vi "EnFlo_Turntable_Control.vi"(3 "Mode":T5=enum."Run VI", 5 "Traverse line In":T2={"Start X"=0.0, "Start Y"=0.0, "Start Z"=0.0, "End X"=0.0, "End Y"=0.0, "End Z"=0.0, "No. of pts."=6, "Spacing"=enum."Linear", "Filename"=path "C:/Enflo_Data_Local/2015/EnFlo_Tunnel/Paul_Hayden/Calibrations/Cal_06-2015/Datum_Block_1.xls", "Tunnel Speed"=0.0, "Averaging time (min)"=0.01, "Extra Commands"="", "Carrier_1 Q (l/min)"=nan, "Carrier_2 Q (l/min)"=nan, "Trace Gas Concentration (%)"=nan, "Specific Arguments"="Datum_Image_Calibration.vi  ", "Comments"="", "Row No"=0, "Row Type Selector"=enum."Run VI Named:", "Completion time"="12:51  12-06-2015", "Row Duration (mins)"=0.11291999999999999, "No. of Valid pts."=6, "Meas Setup File"="Trav_Cam_Picture.xls"} {"Carrier_2 Q (l/min)" format="%#.2f"; "Row Duration (mins)" format="%#.1f"; "Row No" min=0; "Trace Gas Concentration (%)" min=0.0 format="%#_4f"; "Carrier_1 Q (l/min)" format="%#.2f"; "Tunnel Speed" format="%#.2f"; "Start X" format="%#.2f"; "Start Y" format="%#.2f"; "Start Z" format="%#.2f"; "End X" format="%#.2f"; "End Y" format="%#.2f"; "End Z" format="%#.2f"; "Averaging time (min)" min=0.0 format="%#.2f"}) -> (0 "Error Message":string, 1 "Status":T1, 2 "Traverse line Out":T2={"Start X"=0.0, "Start Y"=0.0, "Start Z"=0.0, "End X"=0.0, "End Y"=0.0, "End Z"=0.0, "No. of pts."=6, "Spacing"=enum."Linear", "Filename"=path "C:/Enflo_Data_Local/2015/EnFlo_Tunnel/Paul_Hayden/Calibrations/Cal_06-2015/Datum_Block_1.xls", "Tunnel Speed"=0.0, "Averaging time (min)"=0.01, "Extra Commands"="", "Carrier_1 Q (l/min)"=nan, "Carrier_2 Q (l/min)"=nan, "Trace Gas Concentration (%)"=nan, "Specific Arguments"="Datum_Image_Calibration.vi  ", "Comments"="", "Row No"=0, "Row Type Selector"=enum."Run VI Named:", "Completion time"="12:51  12-06-2015", "Row Duration (mins)"=0.11291999999999999, "No. of Valid pts."=6, "Meas Setup File"="Trav_Cam_Picture.xls"} {"Carrier_2 Q (l/min)" format="%#.2f"; "Row Duration (mins)" format="%#.1f"; "Row No" min=0; "Trace Gas Concentration (%)" min=0.0 format="%#_4f"; "Carrier_1 Q (l/min)" format="%#.2f"; "Tunnel Speed" format="%#.2f"; "Start X" format="%#.2f"; "Start Y" format="%#.2f"; "Start Z" format="%#.2f"; "End X" format="%#.2f"; "End Y" format="%#.2f"; "End Z" format="%#.2f"; "Averaging time (min)" min=0.0 format="%#.2f"})   [LabVIEW 2015]
uses:
  Gen Trav/Traverse_cluster.ctl
  Gen Trav/Spacing.ctl
  Controls/Multi_run_mode.ctl
  Controls/User_Specific_mode.ctl
  Gen Trav/Multi_Run_Status.ctl
  Gen Trav/Trav_mode.ctl
  Controls/Home.ctl
  Controls/Setup.ctl
  Controls/Save_Data.ctl
  ADAM Client/Sub VIs/ADAM Controls/Update_scan_value.ctl
  <vilib>/Analysis/baseanly.llb/Mean (DBL).vi
  Globals/Extra_Commands_Global.vi
  Globals/Trav_pos_global.vi
  Globals/Dynamic_call_global.ph.vi
  <vilib>/Analysis/NI_AALBase.lvlib
panel:
  in  "Ratio of Error to move":dbl=0.75
  in  "stop":bool
  out "Av Meas Angle":dbl format="%0.3f"
  out "Meas Angle":dbl[](array[numeric])
  out "Errors":dbl[](array[numeric])
  in  "Numeric":i32=1
  out "Error in Turntable":dbl(graph)
  in  "Angle Tolerance":dbl=0.01 format="%#_13g"
  out "Turntable Error":dbl
  out "Motor Position (Angle)":dbl(graph)
  out "Demanded Deg":dbl format="%#.4f"
  out "Correct Position":bool
  out "Drive needs relaxing?":bool
  out "Relax Drive":dbl=0.25
  out "+ve Rotation":bool
  out "Motor Current Position":dbl
  # "X           Y            Z"
  # "Start"
  # "End"
  # "X           Y            Z"
  # "Start"
  # "End"
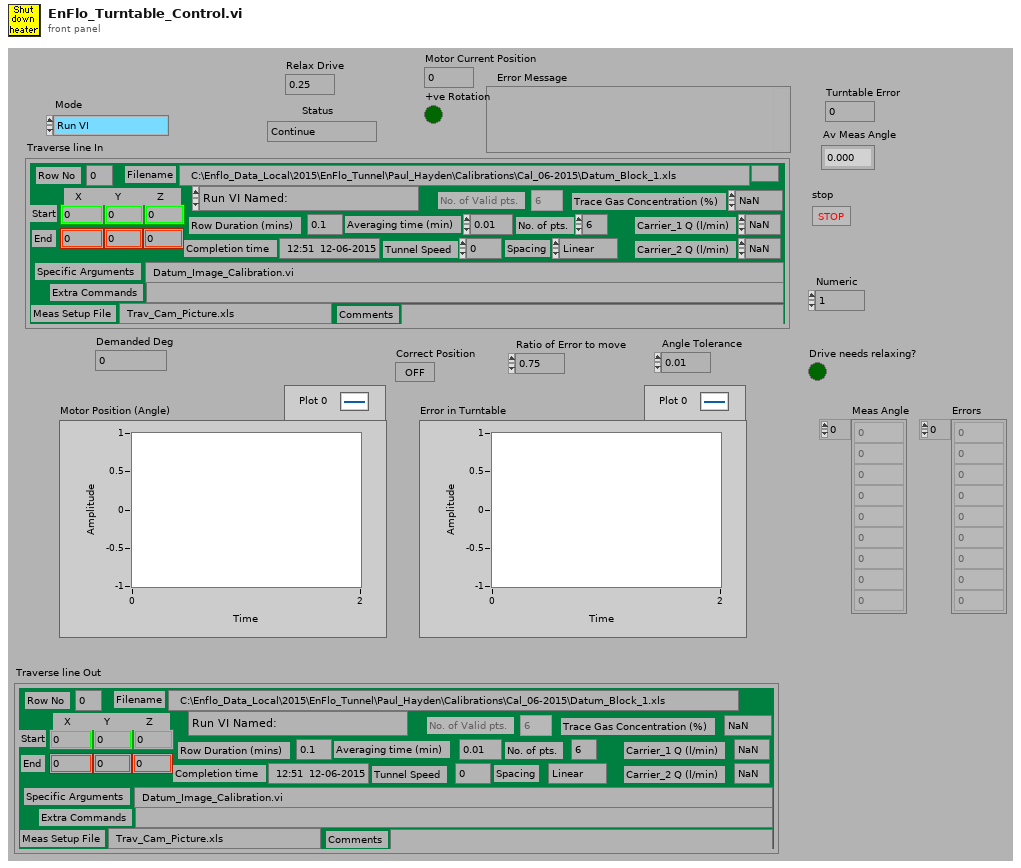
[diagram p1: front panel]
types:
  T1 = typedef "Multi_Run_Status.ctl" = enum16{"Continue", "Jump to Next Point", "Jump to Next Row", "Jump To Fall Back", "Terminate Run"}
  T2 = typedef "Traverse_cluster.ctl" = cluster{"Start X":sgl, "Start Y":sgl, "Start Z":sgl, "End X":sgl, "End Y":sgl, "End Z":sgl, "No. of pts.":i32, "Spacing":T3, "Filename":path, "Tunnel Speed":dbl, "Averaging time (min)":dbl, "Extra Commands":string, "Carrier_1 Q (l/min)":dbl, "Carrier_2 Q (l/min)":dbl, "Trace Gas Concentration (%)":dbl, "Specific Arguments":string, "Comments":string, "Row No":i32, "Row Type Selector":T4, "Completion time":string, "Row Duration (mins)":dbl, "No. of Valid pts.":i32, "Meas Setup File":string}
  T3 = typedef "Spacing.ctl" = enum16{"Linear", "Log", "Gauss", "Specified", "N/A"}
  T4 = typedef "Multi_run_mode.ctl" = enum16{"Move Traverse Only", "Set Tunnel Speed Only", "Set Source Only", "Set Measurement Conditions", "Single Measurement", "Vertical Profile", "Lateral Profile", "Longitudinal Profile", "Explore Volume", "Multi-Axis Profile", "Auto Calibrate", "Meas Fast FID Bkgnd", "Check Beam Power", "Scanning Valve Measurement", "Run VI Named:", "Set ADAM Ch", "Wait (minutes)", "Send Message", "Synchronize With:", "Fall Back to this Row", "Turn Off Row Repeating", "Blank Row", "Traverse 3D Volume"}
  T5 = typedef "User_Specific_mode.ctl" = enum16{"Check VI only", "Run VI"}
  T6 = typedef "Home.ctl" = enum16{"Don't Home", "Home  +X", "Home  -X", "Home  +Y", "Home  -Y", "Home  +Z", "Home  -Z"}
  T7 = typedef "Trav_mode.ctl" = enum16{"Move traverse", "Read traverse position", "Teach Position"}
  T8 = typedef "Save_Data.ctl" = enum16{"Save No Data", "Save Data"}
  T9 = typedef "Setup.ctl" = enum16{"Run Program", "Show Setup", "Save Current Setup", "Setup Front Panel"}
  T10 = typedef "Update_scan_value.ctl" = cluster{"Channel Name":string, "New Value":dbl}
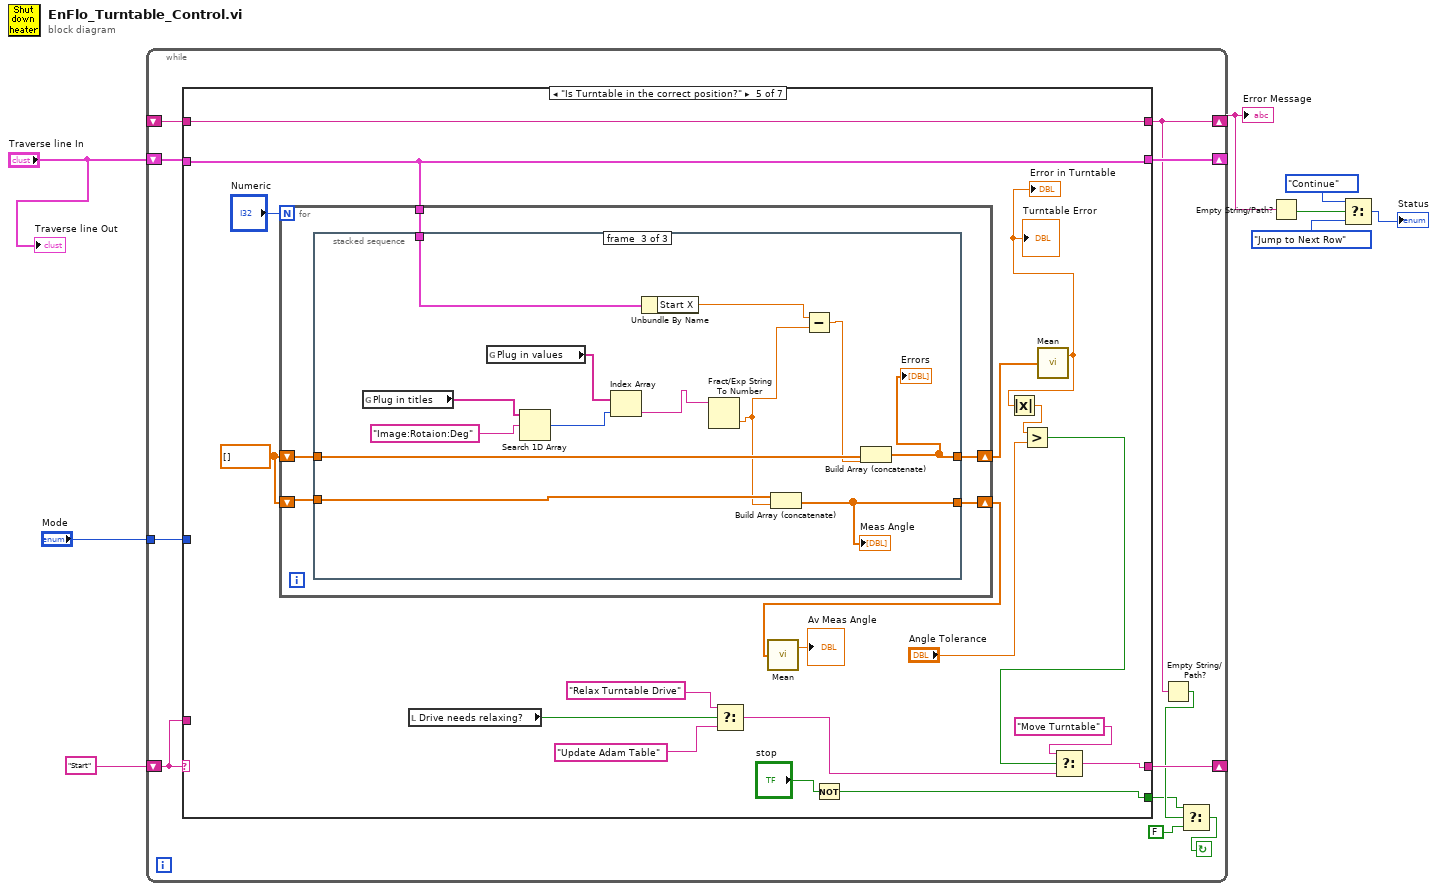
[diagram p0: block diagram]
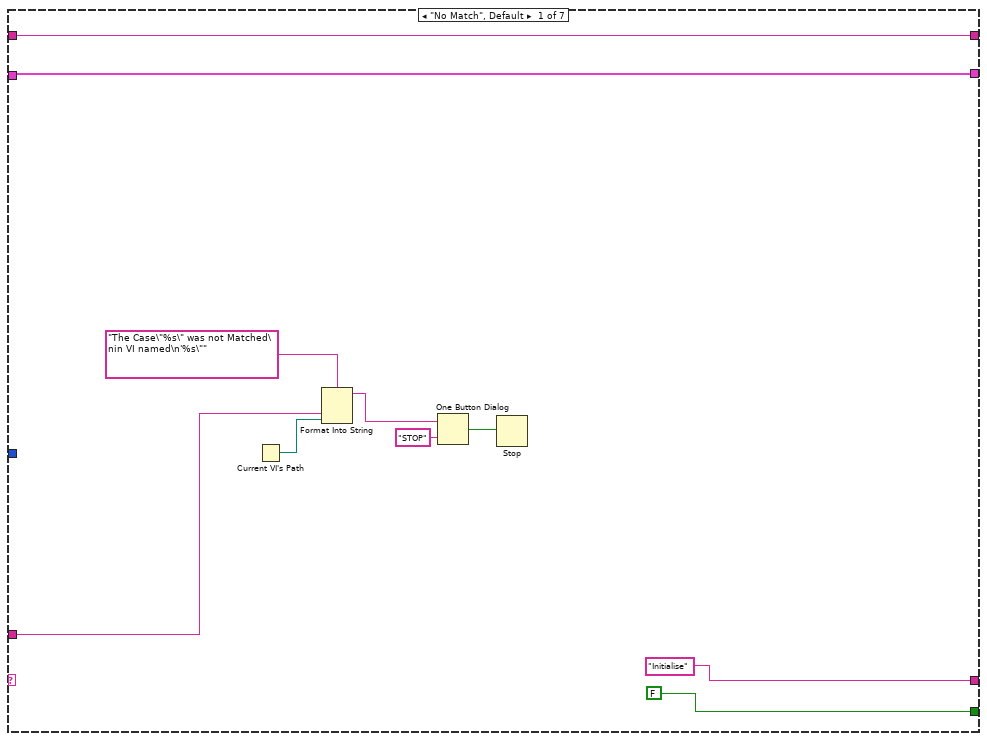
[diagram p2: hidden frame]
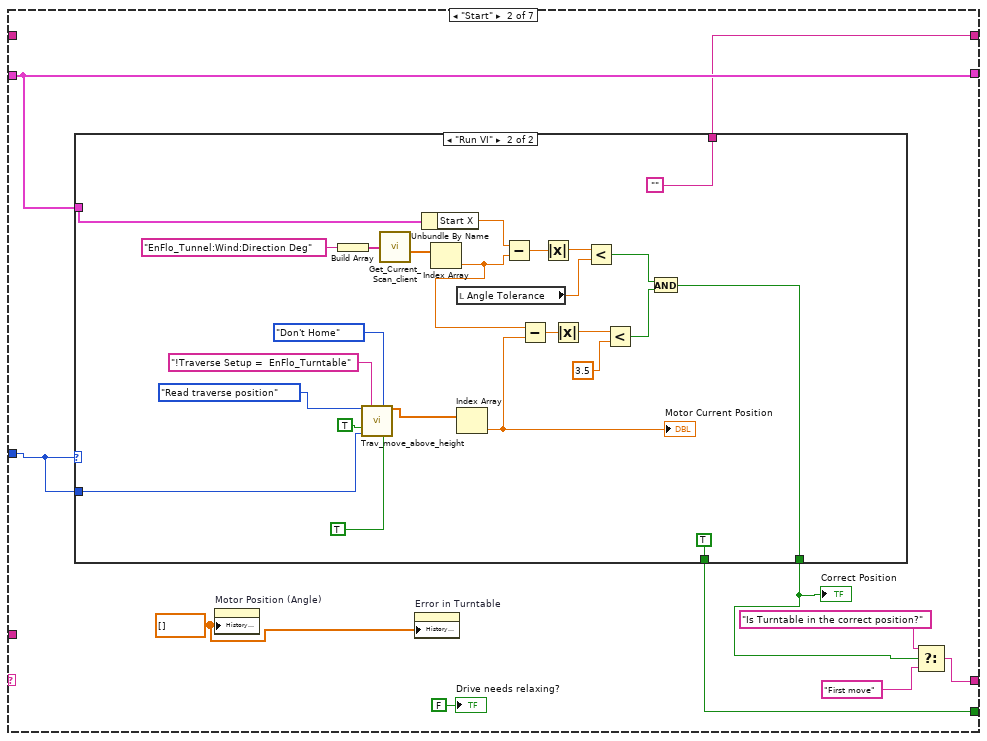
[diagram p3: hidden frame]
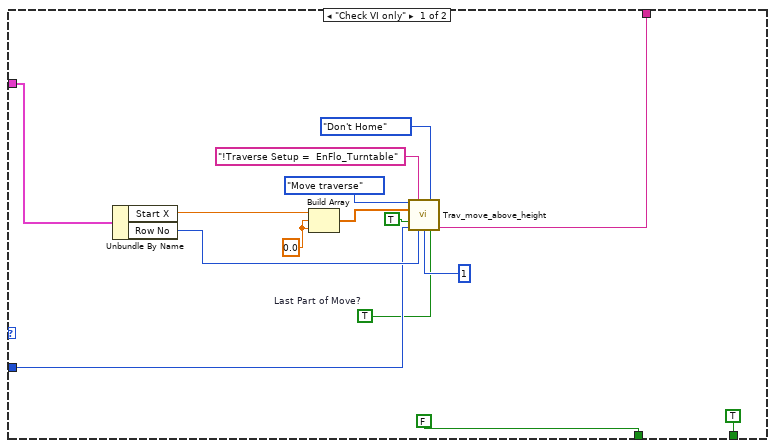
[diagram p4: hidden frame]
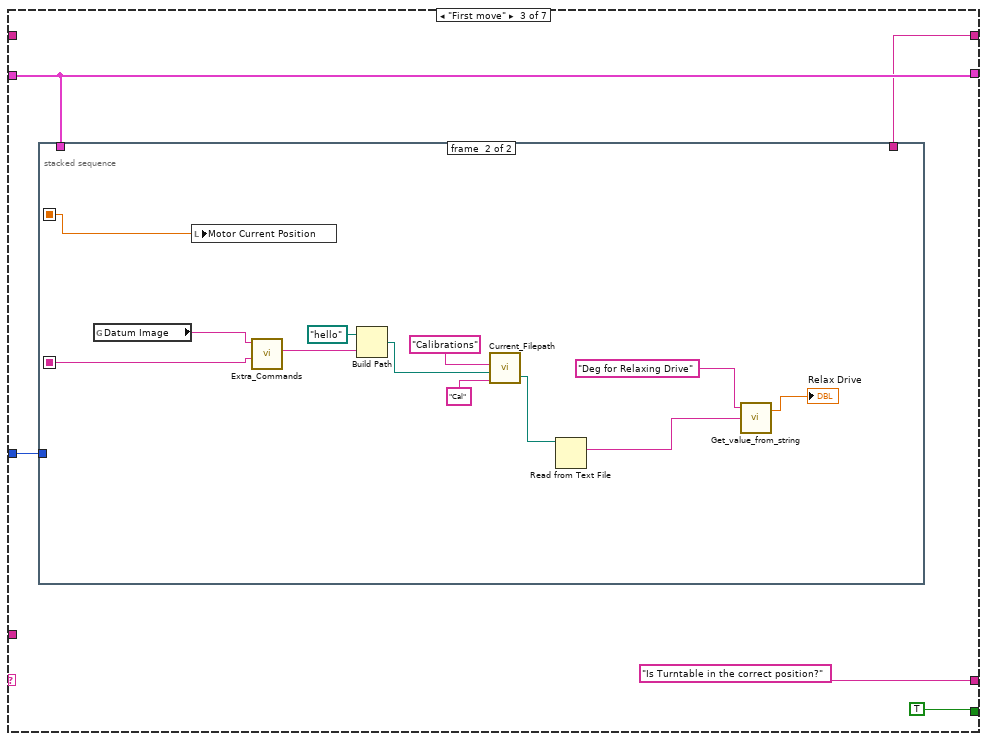
[diagram p5: hidden frame]
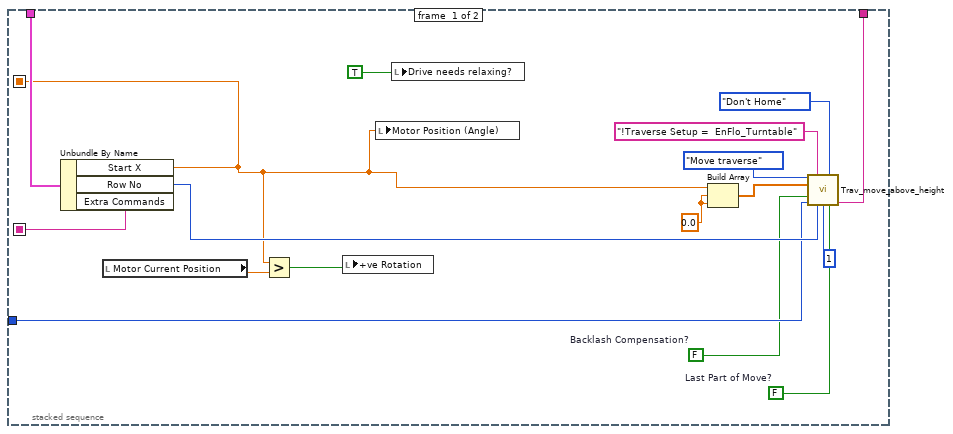
[diagram p6: hidden frame]
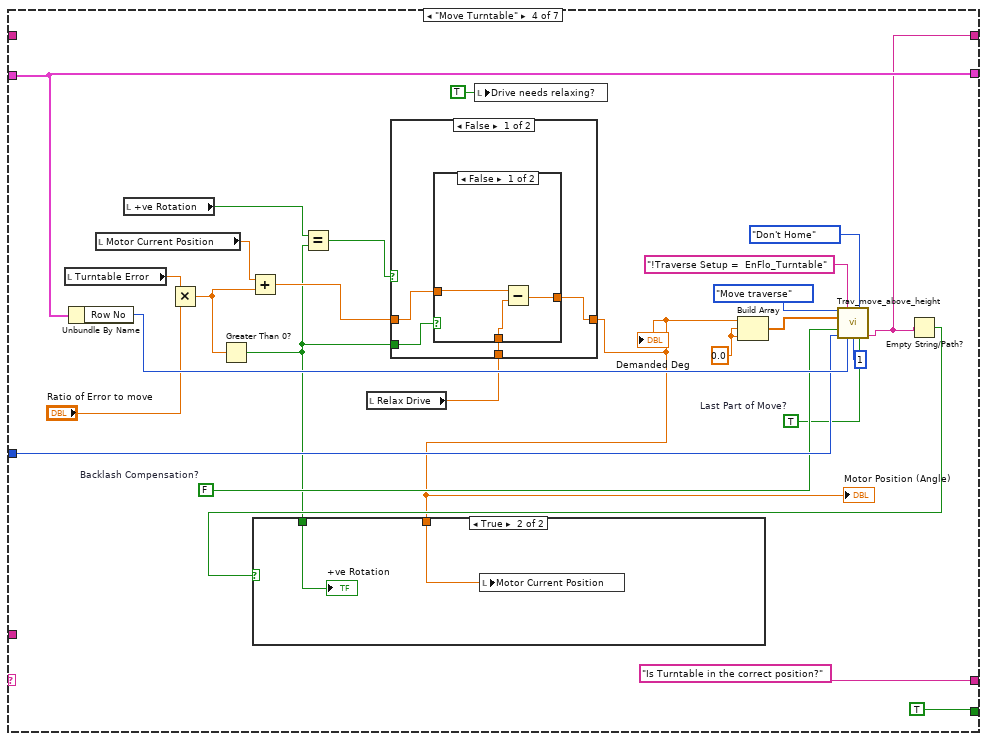
[diagram p7: hidden frame]
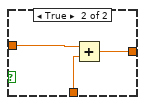
[diagram p8: hidden frame]
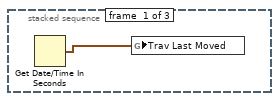
[diagram p11: hidden frame]
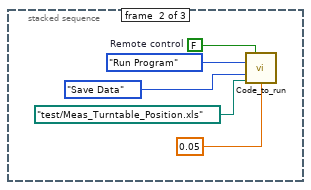
[diagram p12: hidden frame]
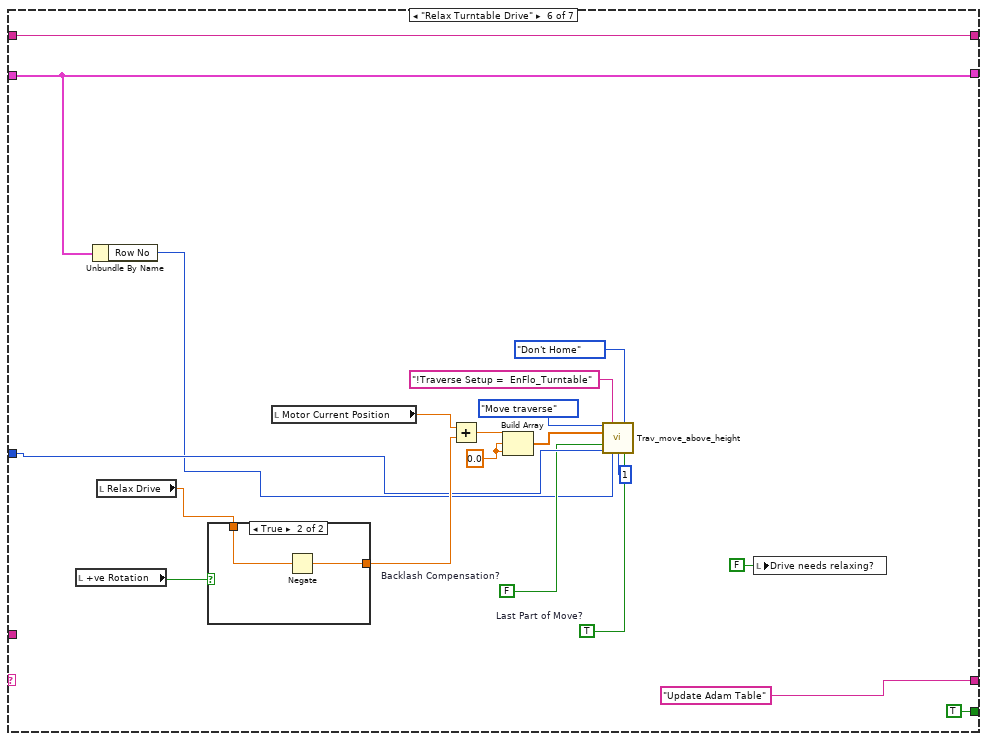
[diagram p13: hidden frame]
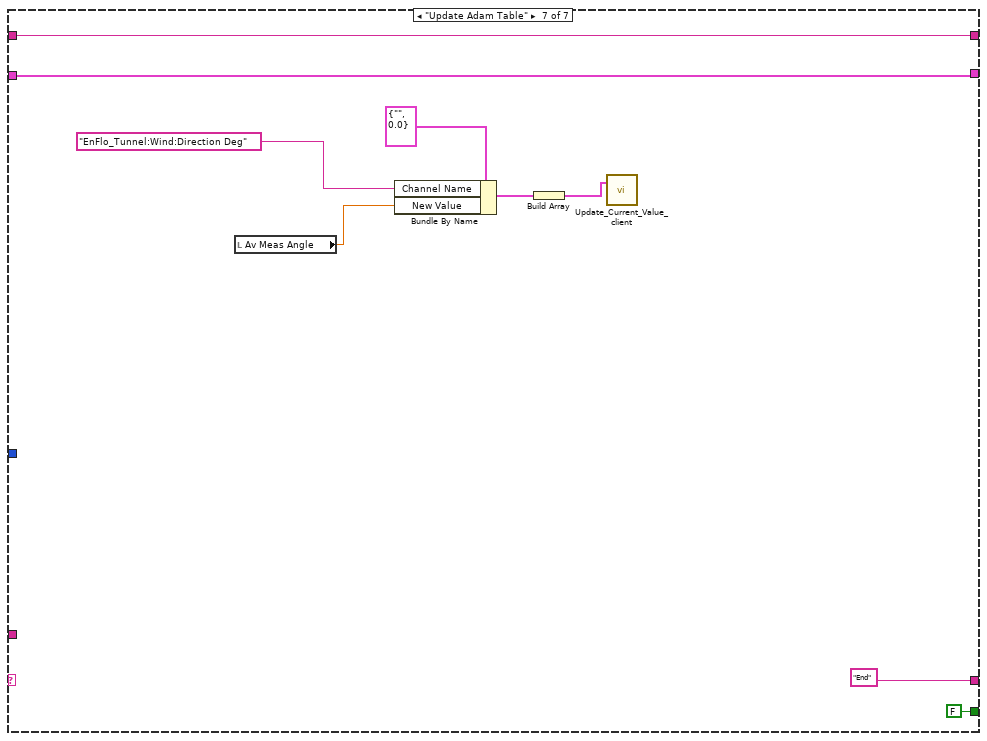
[diagram p15: hidden frame]
diagram:
  n1 = while {
    shift-left: "Start" -> [w18]
    shift-right: [w19] -> _
    tunnel: "Mode" -> [w17]
    shift-right: [w15] -> _
    shift-left: "Traverse line In" -> [w16]
    shift-right: [w13] -> w5
    shift-left: _ -> [w14]
    stop <- w10 continue-if-true
    n2 = case shown="\"Is Turntable in the correct position?\"" w18 {
      tunnel: [FALSE w38 TRUE TRUE w153 TRUE FALSE] -> w11
      tunnel: ["Initialise" w32 "Is Turntable in the correct position?" "Is Turntable in the correct position?" w167 "Update Adam Table" "End"] -> w19
      tunnel: w18 -> [w24 _ _ _ _ _ _]
      tunnel: w17 -> [_ w37 w83 w137 _ w204 _]
      tunnel: w16 -> [w21 w39 w81 w135 w162 w198 w226]
      tunnel: [w21 w39 w81 w135 w162 w198 w226] -> w15
      tunnel: [w20 w36 w80 w127 w171 w215 w221] -> w13
      tunnel: w14 -> [w20 _ _ _ w171 w215 w221]
      frame "No Match", Default {
        n3 = Current VI's Path() -> (path=w23:path)
        n4 = Format Into String(format string="The Case\"%s\" was not Matched\nin VI named\n'%s\"" ("Format String"), w24, w23) -> (resulting string=w27:string)  [unwired: 2 in, 1 out]
        n5 = One Button Dialog(message=w27, button name ("OK")="STOP") -> (true=w25:bool)
        n6 = Stop(stop? (T)=w25) -> ()
      }
      frame "Start" {
        w31 = dbl[] [] ("History Data")
        n7 = case shown="\"Run VI\"" w37 {
          tunnel: w39 -> [w48 w79]
          tunnel: [FALSE TRUE] -> w38
          tunnel: w37 -> [w45 w69]
          tunnel: [w43 ""] -> w36
          tunnel: [TRUE w55] -> w30
          frame "Check VI only" {
            w41 = TRUE  # Last Part of Move?
            w54 = sgl 0.0 ("element")
            n8 = Unbundle By Name(w48) -> ("Start X"=w42:sgl, "Row No"=w47:i32)
            n9 = Build Array(w42, w54, w54) -> (w53:sgl[])
            n10 = call "Trav_move_above_height.vi"("Mode"=Trav_mode."Move traverse", "Extra Command String"="!Traverse Setup =  EnFlo_Turntable", "Home Z"=Home."Don't Home", "New Position"=w53, "Backlash Compensation?"=TRUE, "Simulate/Run"=w45, "Row Number"=w47, "Currently on Point"=1, "Last Part of Move?"=w41) -> ("Error String"=w43:string)  [unwired: 4 in, 2 out]
          }
          frame "Run VI" {
            n11 = Build Array("EnFlo_Tunnel:Wind:Direction Deg") -> (w77:string[])
            n12 = call "Trav_move_above_height.vi"("Mode"=Trav_mode."Read traverse position", "Extra Command String"="!Traverse Setup =  EnFlo_Turntable", "Home Z"=Home."Don't Home", "Backlash Compensation?"=TRUE, "Simulate/Run"=w69, "Last Part of Move?"=TRUE) -> ("Trav Position achieved"=w68:sgl[])  [unwired: 7 in, 2 out]
            n13 = call "Get_Current_Scan_client.vi"("ADAM Ch Names"=w77) -> ("Numerical Values"=w76:dbl[])  [unwired: 1 in, 2 out]
            n14 = Unbundle By Name(w79) -> ("Start X"=w61:sgl)
            n15 = Index Array(array=w76) -> (element=w57:dbl)  [unwired: 1 in]
            n16 = local read "Angle Tolerance"() -> (w58:dbl)
            n17 = Index Array(array=w68) -> (element=w62:sgl)  [unwired: 1 in]
            "Motor Current Position" <- w62
            n18 = Subtract(x=w61, y=w57) -> (x-y=w60:dbl)
            n19 = Subtract(x=w57, y=w62) -> (x-y=w67:dbl)
            n20 = Absolute Value(x=w60) -> (abs(x)=w59:dbl)
            n21 = Absolute Value(x=w67) -> (abs(x)=w66:dbl)
            n22 = Less?(x=w59, y=w58) -> (x < y?=w56:bool)
            n23 = Less?(x=w66, y=sgl 3.5) -> (x < y?=w64:bool)
            n24 = And(x=w56, y=w64) -> (x .and. y?=w55:bool)
          }
        }
        "Correct Position" <- w30
        n25 = property on="Motor Position (Angle)" class="WFChart (strict)"("History Data"=w31) -> ()  [unwired: 2 in, 2 out]
        n26 = property on="Error in Turntable" class="WFChart (strict)"("History Data"=w31) -> ()  [unwired: 2 in, 2 out]
        n27 = Select(t="Is Turntable in the correct position?", s=w30, f="First move") -> (s? t:f=w32:string)
        "Drive needs relaxing?" <- FALSE ("Drive needs relaxing?")
      }
      frame "First move" {
        n28 = stacked-sequence {
          seq-local: [w87 _] -> [_ w113]
          seq-local: [w86 _] -> [_ w102]
          tunnel: w83 -> [w100 _]
          tunnel: w81 -> [w99 _]
          tunnel: [w91 _] -> w80
          frame #0 {
            w90 = FALSE  # Last Part of Move?
            w98 = sgl 0.0 ("element")
            w92 = FALSE  # Backlash Compensation?
            n29 = Unbundle By Name(w99) -> ("Start X"=w87:sgl, "Row No"=w101:i32, "Extra Commands"=w86:string)
            n30 = local read "Motor Current Position"() -> (w89:dbl)
            n31 = Greater?(x=w87, y=w89) -> (0:w88:bool)
            n32 = local write "+ve Rotation"(w88) -> ()
            n33 = local write "Motor Position (Angle)"(w87) -> ()
            n34 = local write "Drive needs relaxing?"(TRUE ("Drive need relaxing?")) -> ()
            n35 = Build Array(w87, w98, w98) -> (w97:sgl[])
            n36 = call "Trav_move_above_height.vi"("Mode"=Trav_mode."Move traverse", "Extra Command String"="!Traverse Setup =  EnFlo_Turntable", "Home Z"=Home."Don't Home", "New Position"=w97, "Backlash Compensation?"=w92, "Simulate/Run"=w100, "Row Number"=w101, "Currently on Point"=1, "Last Part of Move?"=w90) -> ("Error String"=w91:string)  [unwired: 4 in, 2 out]
          }
          frame #1 {
            n37 = global read "Extra_Commands_Global.vi" "Datum Image"() -> (w106:string)
            n38 = local write "Motor Current Position"(w113) -> ()
            n39 = call "Extra_Commands.vi"("String to Search"=w102, "Command"=w106) -> ("String Value"=w111:string)  [unwired: 1 in, 4 out]
            n40 = Build Path(base path=path "hello", name or relative path=w111) -> (appended path=w107:path)
            n41 = call "Current_Filepath.vi"("Short_Name"="Cal" ("Data Type"), "Filename in"=w107, "Data Type"="Calibrations") -> ("Filename Out"=w112:path)  [unwired: 1 in, 1 out]
            n42 = Read from Text File(file (use dialog)=w112) -> (text=w104:string)  [unwired: 3 in, 3 out]
            n43 = call "Get_value_from_string.vi"("Input string"=w104, "Variable name"="Deg for Relaxing Drive" ("Label for characters")) -> ("Value"=→"Relax Drive":dbl)  [unwired: 1 in, 1 out]
          }
        }
      }
      frame "Move Turntable" {
        w124 = TRUE  # Last Part of Move?
        w134 = sgl 0.0 ("element")
        w128 = FALSE  # Backlash Compensation?
        n44 = local read "Turntable Error"() -> (w116:dbl)
        n45 = Unbundle By Name(w135) -> ("Row No"=w138:i32)
        n46 = local read "Motor Current Position"() -> (w123:dbl)
        n47 = local read "+ve Rotation"() -> (w120:bool)
        n48 = Multiply(x=w116, y="Ratio of Error to move") -> (x*y=w114:dbl)
        n49 = Greater Than 0?(x=w114) -> (x > 0?=w118:bool)
        n50 = Add(x=w123, y=w114) -> (x+y=w122:dbl)
        n51 = Equal?(x=w120, y=w118) -> (x = y?=w119:bool)
        n52 = local read "Relax Drive"() -> (w117:dbl)
        n53 = case shown="False" w119 {
          tunnel: w122 -> [w142 w150]
          tunnel: [w141 w150] -> w121
          tunnel: w118 -> [w143 _]
          tunnel: w117 -> [w140 _]
          frame False {
            n54 = case shown="False" w143 {
              tunnel: w142 -> [w146 w149]
              tunnel: [w144 w148] -> w141
              tunnel: w140 -> [w145 w147]
              frame False {
                n55 = Subtract(x=w146, y=w145) -> (x-y=w144:dbl)
              }
              frame True {
                n56 = Add(x=w149, y=w147) -> (x+y=w148:dbl)
              }
            }
          }
          frame True {
          }
        }
        "Demanded Deg" <- w121
        "Motor Position (Angle)" <- w121
        n57 = local write "Drive needs relaxing?"(TRUE ("Drive needs relaxing?")) -> ()
        n58 = Build Array(w121, w134, w134) -> (w133:dbl[])
        n59 = call "Trav_move_above_height.vi"("Mode"=Trav_mode."Move traverse", "Extra Command String"="!Traverse Setup =  EnFlo_Turntable", "Home Z"=Home."Don't Home", "New Position"=w133, "Backlash Compensation?"=w128, "Simulate/Run"=w137, "Row Number"=w138, "Currently on Point"=1, "Last Part of Move?"=w124) -> ("Error String"=w127:string)  [unwired: 4 in, 2 out]
        n60 = Empty String/Path?(string/path=w127) -> (empty?=w126:bool)
        n61 = case shown="True" w126 {
          tunnel: w118 -> [_ w152]
          tunnel: w121 -> [_ w151]
          frame False {
          }
          frame True {
            n62 = local write "Motor Current Position"(w151) -> ()
            "+ve Rotation" <- w152
          }
        }
      }
      frame "Is Turntable in the correct position?" {
        w155 = dbl[] []
        n63 = for {
          N: "Numeric" -> [_]
          tunnel: w162 -> [w176]
          shift-right: [w172] -> w156
          shift-left: w155 -> [w173]
          shift-right: [w174] -> w157
          shift-left: w155 -> [w175]
          n64 = stacked-sequence {
            tunnel: w176 -> [_ _ w190]
            tunnel: w175 -> [_ _ w188]
            tunnel: [_ _ w184] -> w174
            tunnel: w173 -> [_ _ w186]
            tunnel: [_ _ w183] -> w172
            frame #0 {
              n65 = Get Date/Time In Seconds() -> (seconds since 1Jan1904=w177:timestamp)
              n66 = global write "Trav_pos_global.vi" "Trav Last Moved"(w177) -> ()
            }
            frame #1 {
              w182 = FALSE  # Remote control
              n67 = call "Code_to_run.vi"("setup"=Setup."Run Program", "Remote control"=w182, "File"=Save_Data."Save Data", "Results Filename"=path "test/Meas_Turntable_Position.xls", "Averaging time (min)"=0.05) -> ()  [unwired: 6 in, 5 out]
            }
            frame #2 {
              n68 = global read "Dynamic_call_global.ph.vi" "Plug in titles"() -> (w195:string[])
              n69 = global read "Dynamic_call_global.ph.vi" "Plug in values"() -> (w192:string[])
              n70 = Search 1D Array(1D array=w195, element="Image:Rotaion:Deg") -> (index of element=w193:i32)  [unwired: 1 in]
              n71 = Index Array(array=w192, index=w193) -> (element=w191:string)
              n72 = Unbundle By Name(w190) -> ("Start X"=w189:sgl)
              n73 = Fract/Exp String To Number(string=w191) -> (number=w185:dbl)  [unwired: 3 in, 1 out]
              n74 = Build Array (concatenate)(w186, w185) -> (w183:dbl[])
              "Meas Angle" <- w183
              n75 = Subtract(x=w189, y=w185) -> (x-y=w187:dbl)
              n76 = Build Array (concatenate)(w188, w187) -> (w184:dbl[])
              "Errors" <- w184
            }
          }
        }
        n77 = local read "Drive needs relaxing?"() -> (w166:bool)
        n78 = Select(t="Relax Turntable Drive", s=w166, f="Update Adam Table") -> (s? t:f=w165:string)
        n79 = call-poly <vilib>:"Mean.vi"("X"=w156) -> ("mean"=→"Av Meas Angle":dbl)  [unwired: 1 out]
        n80 = Not(x="stop") -> (.not. x?=w153:bool)
        n81 = call-poly <vilib>:"Mean.vi"("X"=w157) -> ("mean"=w159:dbl)  [unwired: 1 out]
        "Turntable Error" <- w159
        "Error in Turntable" <- w159
        n82 = Absolute Value(x=w159) -> (abs(x)=w160:dbl)
        n83 = Greater?(x=w160, y="Angle Tolerance") -> (0:w169:bool)
        n84 = Select(t="Move Turntable", s=w169, f=w165) -> (s? t:f=w167:string)
      }
      frame "Relax Turntable Drive" {
        w199 = TRUE  # Last Part of Move?
        w203 = FALSE  # Backlash Compensation?
        w213 = sgl 0.0 ("element")
        n85 = local read "+ve Rotation"() -> (w207:bool)
        n86 = Unbundle By Name(w198) -> ("Row No"=w197:i32)
        n87 = local read "Relax Drive"() -> (w196:dbl)
        n88 = case shown="True" w207 {
          tunnel: w196 -> [w216 w218]
          tunnel: [w216 w217] -> w205
          frame False {
          }
          frame True {
            n89 = Negate(x=w218) -> (-x=w217:dbl)
          }
        }
        n90 = local read "Motor Current Position"() -> (w201:dbl)
        n91 = Add(x=w201, y=w205) -> (x+y=w206:dbl)
        n92 = Build Array(w206, w213, w213) -> (w212:dbl[])
        n93 = call "Trav_move_above_height.vi"("Mode"=Trav_mode."Move traverse", "Extra Command String"="!Traverse Setup =  EnFlo_Turntable", "Home Z"=Home."Don't Home", "New Position"=w212, "Backlash Compensation?"=w203, "Simulate/Run"=w204, "Row Number"=w197, "Currently on Point"=1, "Last Part of Move?"=w199) -> ()  [unwired: 4 in, 3 out]
        n94 = local write "Drive needs relaxing?"(FALSE ("Drive needs relaxing?")) -> ()
      }
      frame "Update Adam Table" {
        n95 = local read "Av Meas Angle"() -> (w219:dbl)
        n96 = Bundle By Name(cluster=T10 {"Channel Name"="", "New Value"=0.0} ("Update Scan Value Cluster"), "Channel Name"="EnFlo_Tunnel:Wind:Direction Deg", "New Value"=w219) -> (w223:T10)
        n97 = Build Array(w223) -> (w222:T10[])
        n98 = call "Update_Current_Value_client.vi"("Update array in"=w222) -> ()  [unwired: 1 in]
      }
    }
    n99 = Empty String/Path?(string/path=w13) -> (empty?=w12:bool)
    n100 = Select(t=w11, s=w12, f=FALSE) -> (s? t:f=w10:bool)
  }
  "Error Message" <- w5
  n101 = Empty String/Path?(string/path=w5) -> (empty?=w4:bool)
  n102 = Select(t=Multi_Run_Status."Continue" ("Status"), s=w4, f=Multi_Run_Status."Jump to Next Row" ("Status")) -> (s? t:f=→"Status":T1)
  "Traverse line Out" <- "Traverse line In"
